vi "orderbook.test.Delete.Order.First.of.3.vi"(8 "error in":errorcluster) -> (0 "error out":errorcluster, 3 "Passed":bool)   [LabVIEW 2020]
uses:
  arty/orderbook/orderbook.command.ctl
  arty/orderbook/orderbook.command.type.ctl
  arty/application/orderbook.entry.ctl
  arty/application/orderbook.result.type.ctl
panel:
  out "output cluster":T1
  out "OrderBook.Entries":T2[](array[typedef]) {"Side (U8)" format="%.0x"; "Order Id (U64)" format="%.0x"}
  in  "OrderBook.Command[]\nto Send":T4[](array[typedef])=[{"OrderBook Command.Type"=enum."AddOrder", "Side (U8)"=66, "Order Id (U64)"=5129, "Quantity (U32)"=130, "Symbol (U64)"=29033, "Price (U64)"=9525, "Executed Quantity (U32)"=0, "Cancelled Quantity (U32)"=0}, {"OrderBook Command.Type"=enum."AddOrder", "Side (U8)"=66, "Order Id (U64)"=5130, "Quantity (U32)"=225, "Symbol (U64)"=29033, "Price (U64)"=9115, "Executed Quantity (U32)"=0, "Cancelled Quantity (U32)"=0}, {"OrderBook Command.Type"=enum."AddOrder", "Side (U8)"=66, "Order Id (U64)"=5131, "Quantity (U32)"=50, "Symbol (U64)"=29033, "Price (U64)"=9200, "Executed Quantity (U32)"=0, "Cancelled Quantity (U32)"=0}, {"OrderBook Command.Type"=enum."DeleteOrder", "Side (U8)"=0, "Order Id (U64)"=5130, "Quantity (U32)"=0, "Symbol (U64)"=0, "Price (U64)"=0, "Executed Quantity (U32)"=0, "Cancelled Quantity (U32)"=0}, {"OrderBook Command.Type"=enum."Get.All.Orders", "Side (U8)"=0, "Order Id (U64)"=0, "Quantity (U32)"=0, "Symbol (U64)"=0, "Price (U64)"=0, "Executed Quantity (U32)"=0, "Cancelled Quantity (U32)"=0}] {"Side (U8)" format="%.0x"; "Order Id (U64)" format="%.0x"; "Symbol (U64)" format="%.0x"}
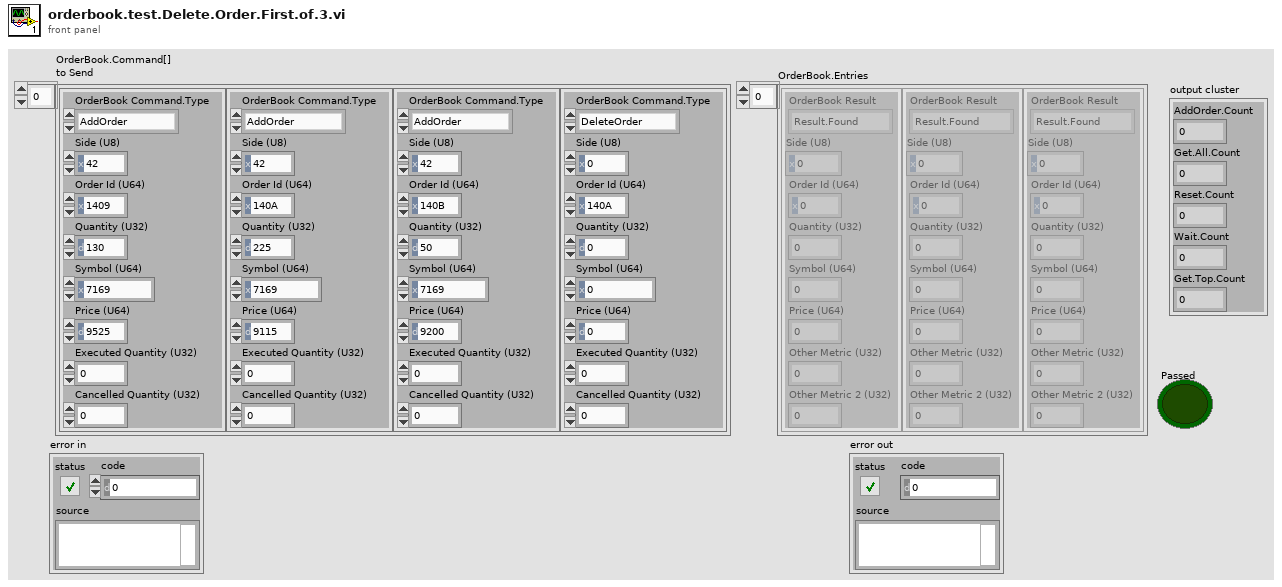
[diagram p1: front panel]
types:
  T1 = cluster{"AddOrder.Count":u32, "Get.All.Count":u32, "Reset.Count":u32, "Wait.Count":u32, "Get.Top.Count":u32}
  T2 = typedef "orderbook.entry.ctl" = cluster{"OrderBook Result":T3, "Side (U8)":u8, "Order Id (U64)":u64, "Quantity (U32)":u32, "Symbol (U64)":u64, "Price (U64)":u64, "Other Metric (U32)":u32, "Other Metric 2 (U32)":u32}
  T3 = typedef "orderbook.result.type.ctl" = enum16{"Result.Found", "Result.Not.Found"}
  T4 = typedef "orderbook.command.ctl" = cluster{"OrderBook Command.Type":T5, "Side (U8)":u8, "Order Id (U64)":u64, "Quantity (U32)":u32, "Symbol (U64)":u64, "Price (U64)":u64, "Executed Quantity (U32)":u32, "Cancelled Quantity (U32)":u32}
  T5 = typedef "orderbook.command.type.ctl" = enum16{"AddOrder", "OrderExecuted", "ReduceSize", "ModifyOrder", "DeleteOrder", "Get.All.Orders", "Get.Top"}
  T6 = cluster{"Write.Request":bool, "Read.Request":bool, "Read.Address":u32, "Read.OrderBook.Entry":cluster{"OrderBook Result":enum16{"Result.Found", "Result.Not.Found"}, "Side (U8)":u8, "Order Id (U64)":u64, "Quantity (U32)":u32, "Symbol (U64)":u64, "Price (U64)":u64, "Other Metric (U32)":u32, "Other Metric 2 (U32)":u32}, "Number.of.Entries":u32, "OrderBook.State":enum16{"Reset", "WaitForNewCommand", "AddOrder", "Get.All.Orders", "Get.Top"}, "Ready.For.OrderBook.Command":bool, "Memory.State":enum16{"New", "Request.Data", "Append", "Data.Ready"}, "Move":bool, "Read.Valid":bool, "Write.Address":u32, "Write.OrderBook.Entry":cluster{"OrderBook Result":enum16{"Result.Found", "Result.Not.Found"}, "Side (U8)":u8, "Order Id (U64)":u64, "Quantity (U32)":u32, "Symbol (U64)":u64, "Price (U64)":u64, "Other Metric (U32)":u32, "Other Metric 2 (U32)":u32}, "OrderBook.Result.Valid":bool, "AddOrder.Count":u32, "Get.All.Count":u32, "Reset.Count":u32, "Wait.Count":u32, "Append":bool, "Get.Top.Count":u32}
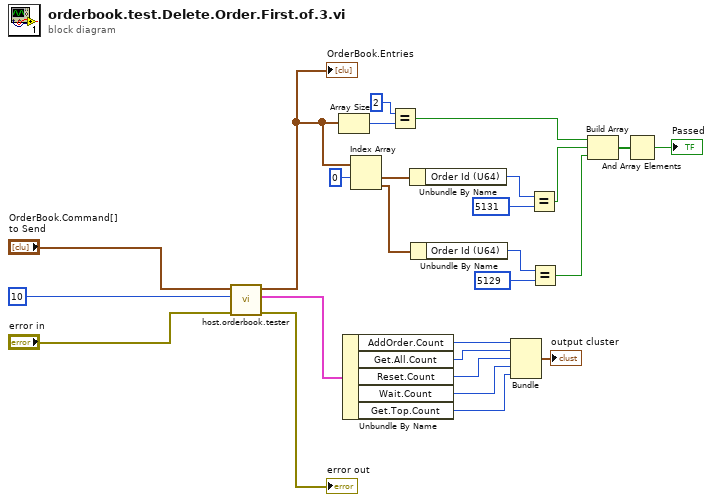
[diagram p0: block diagram]
diagram:
  n1 = call "host.orderbook.tester.vi"("error in"="error in", "Seconds to Wait"=10 ("Seconds\nto\nWait"), "OrderBook.Command[]\nto Send"="OrderBook.Command[]\nto Send") -> ("error out"=→"error out":errorcluster, "OrderBook.Variables"=w10:T6, "OrderBook.Entries"=w8:T2[])  [unwired: 6 in]
  "OrderBook.Entries" <- w8
  n2 = Array Size(array=w8) -> (size(s)=w19:i32)
  n3 = Unbundle By Name(w10) -> ("AddOrder.Count"=w23:u32, "Get.All.Count"=w20:u32, "Reset.Count"=w21:u32, "Wait.Count"=w22:u32, "Get.Top.Count"=w6:u32)
  n4 = Index Array(array=w8, index #1=0 ("index")) -> (element #1=w17:T2, element #2=w2:T2)  [unwired: 1 in]
  n5 = Equal?(x=2, y=w19) -> (x = y?=w13:bool)
  n6 = Unbundle By Name(w17) -> ("Order Id (U64)"=w15:u64)
  n7 = Unbundle By Name(w2) -> ("Order Id (U64)"=w4:u64)
  n8 = Bundle("AddOrder.Count"=w23, "Get.All.Count"=w20, "Reset.Count"=w21, "Wait.Count"=w22, "Get.Top.Count"=w6) -> (→"output cluster":T1)  [unwired: 1 in]
  n9 = Equal?(x=w15, y=u64 5131) -> (x = y?=w14:bool)
  n10 = Equal?(x=w4, y=u64 5129) -> (x = y?=w1:bool)
  n11 = Build Array(w13, w14, w1) -> (w12:bool[])
  n12 = And Array Elements(Boolean array=w12) -> (logical AND=→"Passed":bool)
